vi "set_value.vi"(8 "error in (no error)":errorcluster, 10 "value":T1, 11 "Dimension in":refnum<class "Dimension.lvclass">) -> (0 "error out":errorcluster, 3 "Dimension out":refnum<class "Dimension.lvclass">)   [LabVIEW 2020, in "mlir.lvlib" / "Dimension.lvclass"]
uses:
  Dimension.lvclass
  Dimension.lvclass/Dimension.ctl
  value.ctl
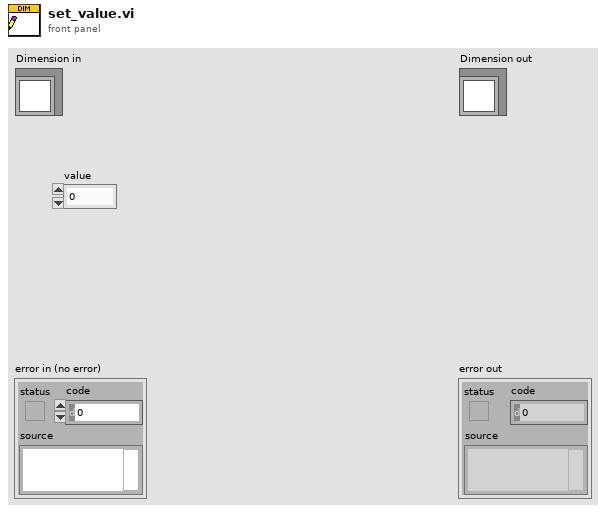
[diagram p1: front panel]
types:
  T1 = typedef "mlir.lvlib/Dimension.lvclass/value.ctl" = u32
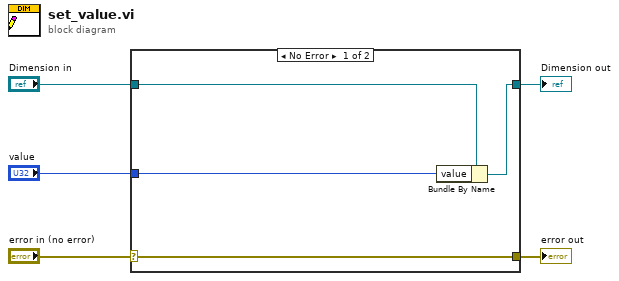
[diagram p0: block diagram]
diagram:
  n1 = case shown="No Error" "error in (no error)" {
    selector: "error in (no error)" -> [w9 w10]
    tunnel: [w9 w10] -> w4
    tunnel: [w7 w11] -> w2
    tunnel: "Dimension in" -> [w8 w11]
    tunnel: "value" -> [w6 _]
    frame No Error {
      n2 = Bundle By Name(cluster=w8, "value"=w6) -> (w7:refnum<class "Dimension.lvclass">)
    }
    frame Error {
    }
  }
  "error out" <- w4
  "Dimension out" <- w2
